vi "mxwScript_API_SetVal_LoneXNodeState.vi"(8 "error in (no error)":errorcluster, 11 "XNode state":T2) -> (0 "error out":errorcluster, 3 "parameter":T1)   [LabVIEW 2020]
uses:
  codeGenAPISupport.llb/cgAPI_mxwScript_XNodeState.ctl
  codeGenAPISupport.llb/cgAPI_mxwScript_VersionInfo.ctl
  codeGenAPISupport.llb/cgAPI_mxwScript_Parameter.ctl
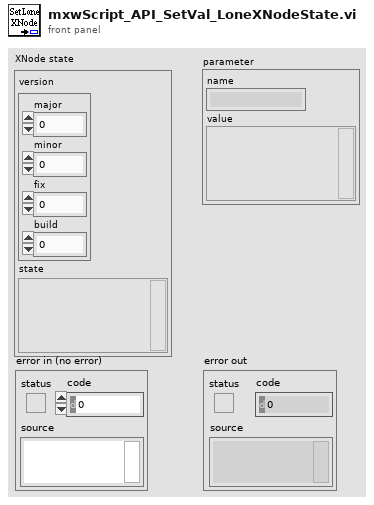
[diagram p1: front panel]
types:
  T1 = typedef "cgAPI_mxwScript_Parameter.ctl" = cluster{"name":string, "value":variant}
  T2 = typedef "cgAPI_mxwScript_XNodeState.ctl" = cluster{"version":T3, "state":variant}
  T3 = typedef "cgAPI_mxwScript_VersionInfo.ctl" = cluster{"major":u16, "minor":u16, "fix":u16, "build":u16}
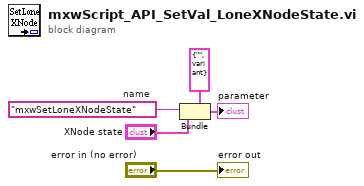
[diagram p0: block diagram]
diagram:
  w2 = "mxwSetLoneXNodeState"  # name
  n1 = Bundle(cluster=T1 {"name"="", "value"=variant} ("parameter"), "name"=w2, "value"="XNode state") -> (→"parameter":T1)
  "error out" <- "error in (no error)"
